vi "Pull data from disc.vi"(8 "error in":errorcluster, 10 "Graphic Root Folder":path, 11 "Data in":T1[](array[typedef])) -> (0 "error out":errorcluster, 3 "Data out":T1[](array[typedef]))   [LabVIEW 2021]
uses:
  <resource>/plugins/NIIconEditor/Controls/IconFilename.ctl
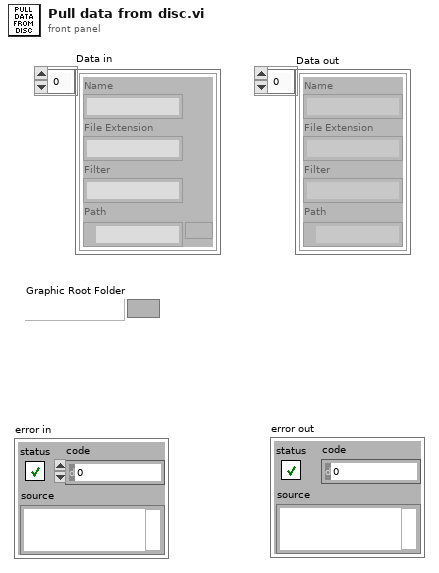
[diagram p1: front panel]
types:
  T1 = typedef "IconFilename.ctl" = cluster{"Name":string, "File Extension  ":string, "Filter":string, "Path":path}
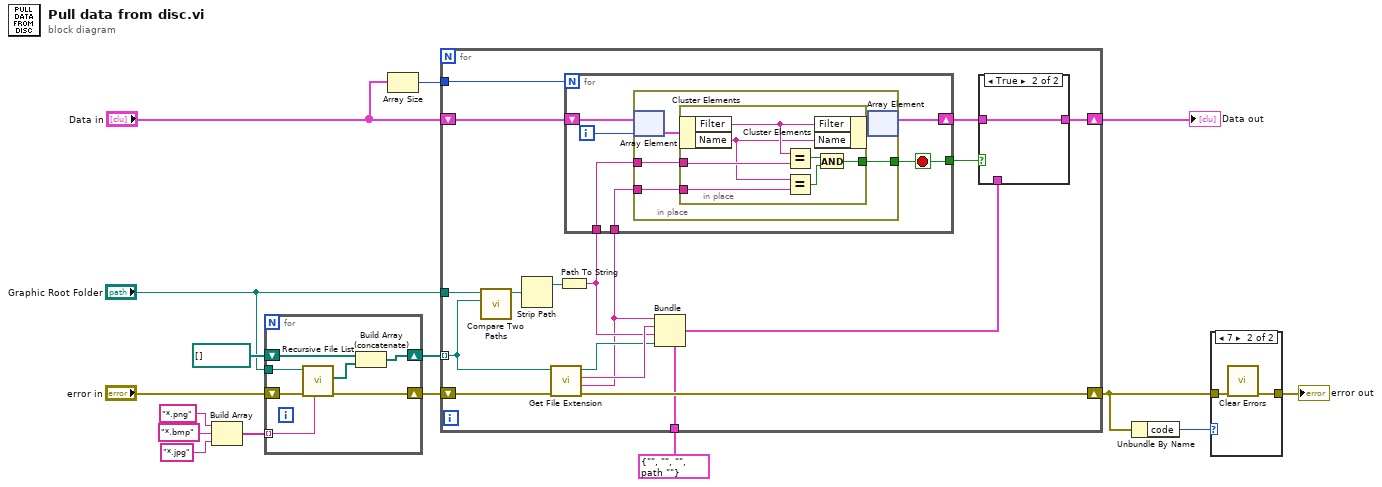
[diagram p0: block diagram]
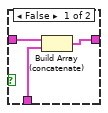
[diagram p3: hidden frame]
diagram:
  n1 = Build Array("*.png" ("pattern"), "*.bmp" ("pattern"), "*.jpg" ("pattern")) -> (w13:string[])
  n2 = for {
    tunnel: "Graphic Root Folder" -> [w23]
    shift-right: [w21] -> w15
    shift-left: path[] [] -> [w20]
    tunnel: w13 -> [w22] mode=indexing
    shift-right: [w17] -> w16
    shift-left: "error in" -> [w18]
    n3 = call <vilib>:"Recursive File List.vi"("pattern"=w22, "error in (no error)"=w18, "Folder Path"=w23) -> ("error out"=w17:errorcluster, "All Files in Dir"=w19:path[])  [unwired: 1 in, 6 out]
    n4 = Build Array (concatenate)(w20, w19) -> (w21:path[])
  }
  n5 = Array Size(array="Data in") -> (size(s)=w6:i32)
  n6 = for {
    tunnel: w15 -> [w35] mode=indexing
    shift-right: [w37] -> w2
    shift-left: w16 -> [w40]
    tunnel: "Graphic Root Folder" -> [w36]
    tunnel: T1 {"Name"="", "File Extension  "="", "Filter"="", "Path"=path ""} ("cluster") -> [w32]
    shift-right: [w25] -> w5
    shift-left: "Data in" -> [w31]
    tunnel: w6 -> [w30]
    n7 = call <vilib>:"Compare Two Paths.vi"("Path 2"=w35, "Path 1"=w36) -> ("Relative Path from 1 to 2"=w33:path)  [unwired: 1 in, 8 out]
    n8 = Strip Path(path=w33) -> (stripped path=w34:path)  [unwired: 1 out]
    n9 = call <vilib>:"Get File Extension.vi"("error in (no error)"=w40, "file"=w35) -> ("error out"=w37:errorcluster, "filename without extension"=w24:string, "lowercase file extension"=w39:string, "dup file"=w38:path)  [unwired: 6 out]
    n10 = Path To String(path=w34) -> (string=w29:string)
    n11 = for {
      N: w30 -> [_]
      shift-right: [w48] -> w27
      shift-left: w31 -> [w50]
      tunnel: w29 -> [w47]
      tunnel: [w46] -> w28
      tunnel: w24 -> [w45]
      i -> [w49]
      stop <- w46 stop-if-true
      n12 = in-place {
        in-place-border: w47 -> [w54]
        in-place-border: [w52] -> w46
        in-place-border: w45 -> [w51]
        n13 = in-place-array #1(w50, w49) -> (w55:T1)
        n14 = in-place {
          in-place-border: w54 -> [w62]
          in-place-border: [w57] -> w52
          in-place-border: w51 -> [w60]
          n15 = in-place-cluster #2(w55) -> ("Filter"=w61:string, "Name"=w56:string)
          n16 = Equal?(x=w61, y=w62) -> (x = y?=w59:bool)
          n17 = Equal?(x=w56, y=w60) -> (x = y?=w58:bool)
          n18 = in-place-cluster #2("Filter"=w61, "Name"=w56) -> (w53:T1)
          n19 = And(x=w59, y=w58) -> (x .and. y?=w57:bool)
        }
        n20 = in-place-array #1(w53) -> (w48:T1[])  [unwired: 1 out]
      }
    }
    n21 = Bundle(cluster=w32, "Name"=w24, "File Extension"=w39, "Filter"=w29, "Path"=w38) -> (w26:T1)
    n22 = case shown="True" w28 {
      tunnel: w27 -> [w43 w44]
      tunnel: w26 -> [w42 _]
      tunnel: [w41 w44] -> w25
      frame False {
        n23 = Build Array (concatenate)(w43, w42) -> (w41:T1[])
      }
      frame True {
      }
    }
  }
  "Data out" <- w5
  n24 = Unbundle By Name(w2) -> ("code"=w3:i32)
  n25 = case shown="7" w3 {
    tunnel: w2 -> [w63 w65]
    tunnel: [w63 w64] -> w1
    frame 0, Default {
    }
    frame 7 {
      n26 = call <vilib>:"Clear Errors.vi"("error in (no error)"=w65) -> ("error out"=w64:errorcluster)  [unwired: 1 in, 5 out]
    }
  }
  "error out" <- w1
